vi "TimeScale.vi"(7 "Variables":T1={"Boltzmans "=1.3806e-23, "Temp K"=293.0, "Viscosity"=0.00089, "lamda (m)"=6.4e-07, "n"=1.33}, 10 "Diameter (m)":dbl, 11 "Angle (degrees)":dbl=90.0) -> (2 "Theory":T2)   [LabVIEW 2022 SP3]
panel:
  out "q":dbl
  out "D":dbl
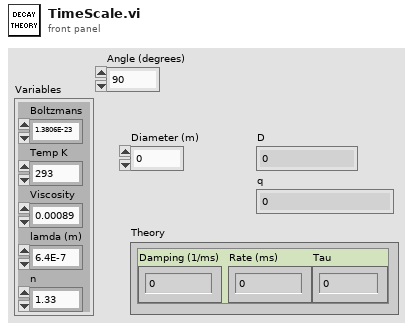
[diagram p1: front panel]
types:
  T1 = cluster{"Boltzmans ":dbl, "Temp K":dbl, "Viscosity":dbl, "lamda (m)":dbl, "n":dbl}
  T2 = cluster{"Damping (1/ms)":dbl, "Rate (ms)":dbl, "Tau":dbl}
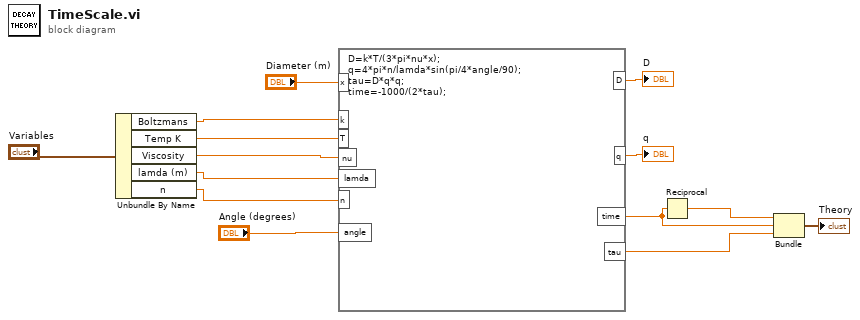
[diagram p0: block diagram]
diagram:
  n1 = Unbundle By Name("Variables") -> ("Boltzmans"=w5:dbl, "Temp K"=w6:dbl, "Viscosity"=w4:dbl, "lamda (m)"=w3:dbl, "n"=w2:dbl)
  n2 = formula code="D=k*T/(3*pi*nu*x);\nq=4*pi*n/lamda*sin(pi/4*angle/90);\ntau=D*q*q;\ntime=-1000/(2*tau);"("k"=w5, "T"=w6, "nu"=w4, "lamda"=w3, "n"=w2, "x"="Diameter (m)", "angle"="Angle (degrees)") -> ("D"=→"D":dbl, "q"=→"q":dbl, "time"=w8:dbl, "tau"=w12:dbl)
  n3 = Reciprocal(x=w8) -> (1/x=w10:dbl)
  n4 = Bundle(w10, "time"=w8, "tau"=w12) -> (→"Theory":cluster{dbl, "time":dbl, "tau":dbl})  [unwired: 1 in]
